vi "Troubleshoot 1.vi"(8 "error in (no error)":errorcluster, 9 "Network Settings in":T6, 10 "Targets in":T1 {"Filtered Targets"."IP Mode" items=["Static"=1, "DHCP/Link-Local"=2, "Link-Local Only"=4, "DHCP Only"=8]}, 11 "Ctl Refs in":T7) -> (0 "error out":errorcluster, 1 "Network Settings out":T6, 2 "Targets out":T1 {"Filtered Targets"."IP Mode" items=["Static"=1, "DHCP/Link-Local"=2, "Link-Local Only"=4, "DHCP Only"=8]}, 3 "Ctl Refs out":T7, 4 "Buttons out":T5, 5 "Execution State":T4, 7 "Deploy out":enum16{"Deploy", "Troubleshoot"}(ring))   [LabVIEW 2013]
uses:
  Controls/Refs.ctl
  Controls/Button Refs.ctl
  Controls/Tab Ctl Refs.ctl
  types/TabStateType.ctl
  Controls/Indicator Refs.ctl
  Controls/Slider Refs.ctl
  Controls/Control Refs.ctl
  Controls/Targets.ctl
  Controls/Detected.ctl
  types/MAX Sys Cfg Target Information.ctl
  Controls/Network Settings.ctl
  types/ButtonStateType.ctl
  types/ExecutionStateType.ctl
panel:
  in  "stop_loop":bool
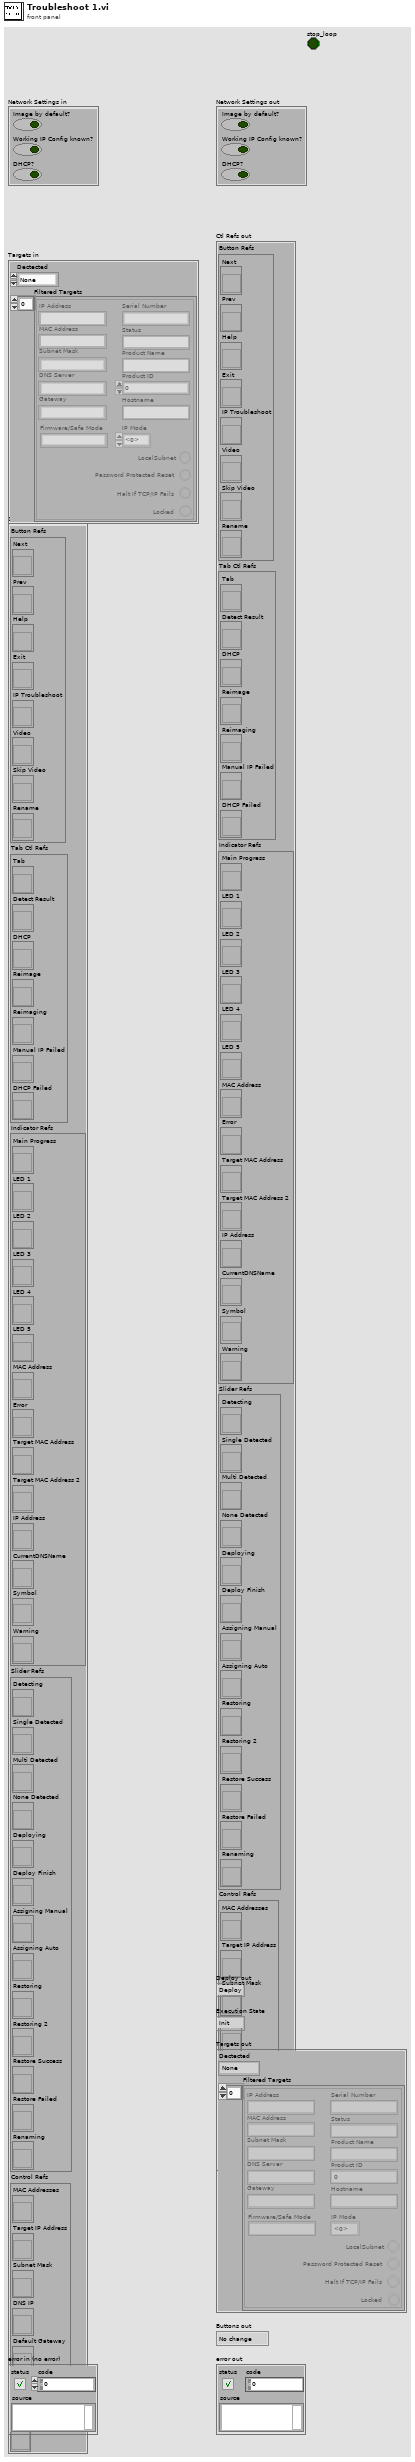
[diagram p1: front panel]
types:
  T1 = typedef "Targets.ctl" = cluster{"Dectected":T2, "Filtered Targets":T3[]}
  T2 = typedef "Detected.ctl" = enum16{"None", "Failed", "Single", "Multi"}
  T3 = typedef "MAX Sys Cfg Target Information.ctl" = cluster{"MAC Address":string, "IP Address":string, "Status":string, "Product Name":string, "Hostname":string, "Firmware/Safe Mode":string, "Subnet Mask":string, "Gateway":string, "DNS Server":string, "Serial Number":string, "Product ID":u32, "Locked ":bool, "LocalSubnet":bool, "Halt If TCP/IP Fails":bool, "Password Protected Reset":bool, "IP Mode":i32}
  T4 = typedef "ExecutionStateType.ctl" = enum16{"Init", "Welcome", "Idle", "Detect", "Run Detection", "Detect Fail", "Detect One", "Detect Mult", "Deploy", "DHCP", "Static IP", "Run Deployment", "Connect Verify", "Exit", "Video Wait", "Success", "Troubleshoot", "Troubleshoot 2", "RenameDNS"}
  T5 = typedef "ButtonStateType.ctl" = enum16{"No change", "No Next", "No Prev", "All Disabled", "All Enabled", "Exit Only"}
  T6 = typedef "Network Settings.ctl" = cluster{"Image by default?":bool, "Working IP Config known?":bool, "DHCP?":bool}
  T7 = typedef "Refs.ctl" = cluster{"Button Refs":T8, "Tab Ctl Refs":T9, "Indicator Refs":T10, "Slider Refs":T11, "Control Refs":T12, "Deploy Message":refnum<vi>}
  T8 = typedef "Button Refs.ctl" = cluster{"Next":refnum<vi>, "Prev":refnum<vi>, "Help":refnum<vi>, "Exit":refnum<vi>, "IP Troubleshoot":refnum<vi>, "Video":refnum<vi>, "Skip Video":refnum<vi>, "Rename":refnum<vi>}
  T9 = typedef "Tab Ctl Refs.ctl" = cluster{"Tab":refnum<vi>, "Detect Result":refnum<vi>, "DHCP":refnum<vi>, "Reimage":refnum<vi>, "Reimaging":refnum<vi>, "Manual IP Failed":refnum<vi>, "DHCP Failed":refnum<vi>}
  T10 = typedef "Indicator Refs.ctl" = cluster{"Main Progress":refnum<vi>, "LED 1":refnum<vi>, "LED 2":refnum<vi>, "LED 3":refnum<vi>, "LED 4":refnum<vi>, "LED 5":refnum<vi>, "MAC Address":refnum<vi>, "Error":refnum<vi>, "Target MAC Address":refnum<vi>, "Target MAC Address 2":refnum<vi>, "IP Address":refnum<vi>, "CurrentDNSName":refnum<vi>, "Symbol":refnum<vi>, "Warning":refnum<vi>}
  T11 = typedef "Slider Refs.ctl" = cluster{"Detecting":refnum<vi>, "Single Detected":refnum<vi>, "Multi Detected":refnum<vi>, "None Detected":refnum<vi>, "Deploying":refnum<vi>, "Deploy Finish":refnum<vi>, "Assigning Manual":refnum<vi>, "Assigning Auto":refnum<vi>, "Restoring":refnum<vi>, "Restoring 2":refnum<vi>, "Restore Success":refnum<vi>, "Restore Failed":refnum<vi>, "Renaming":refnum<vi>}
  T12 = typedef "Control Refs.ctl" = cluster{"MAC Addresses":refnum<vi>, "Target IP Address":refnum<vi>, "Subnet Mask":refnum<vi>, "DNS IP":refnum<vi>, "Default Gateway":refnum<vi>, "DNSName":refnum<vi>}
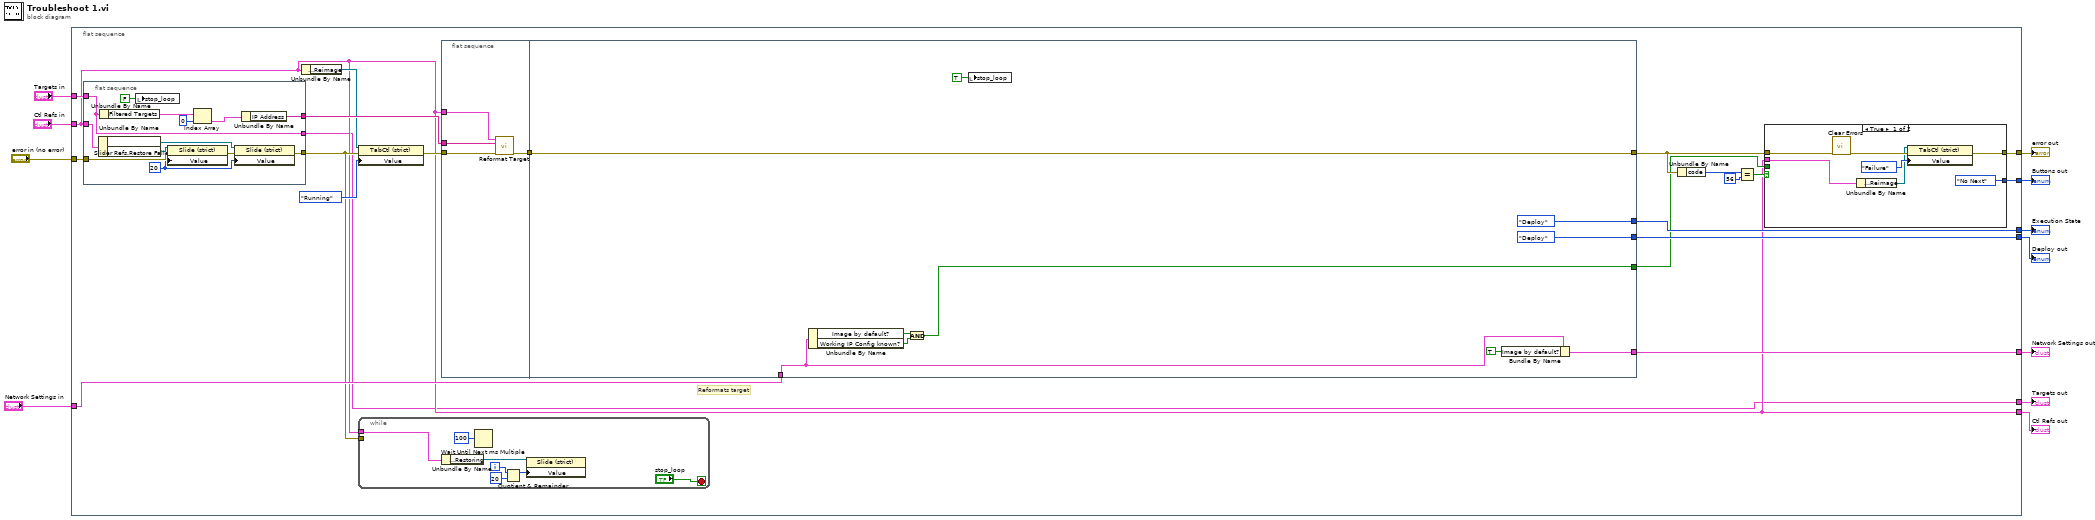
[diagram p0: block diagram]
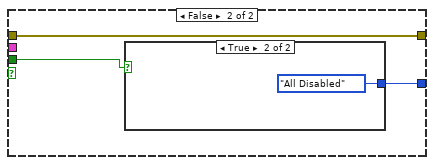
[diagram p2: hidden frame]
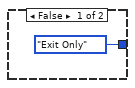
[diagram p3: hidden frame]
diagram:
  n1 = flat-sequence {
    tunnel: "Targets in" -> [w31]
    tunnel: "error in (no error)" -> [w30]
    tunnel: [w26] -> w3
    tunnel: [w25] -> w4
    tunnel: [w20] -> w5
    tunnel: [w19] -> w6
    tunnel: "Network Settings in" -> [w18]
    tunnel: [w15] -> w8
    tunnel: [w12] -> w9
    tunnel: "Ctl Refs in" -> [w13]
    tunnel: [w13] -> w11
    frame #0 {
      # "Reformats target"
      n2 = flat-sequence {
        tunnel: w31 -> [w75]
        tunnel: [w75] -> w12
        tunnel: [w67] -> w16
        tunnel: w30 -> [w73]
        tunnel: [w76] -> w27
        tunnel: w13 -> [w70]
        frame #0 {
          w71 = i8 20 ("Slide 9")
          n3 = Unbundle By Name(w70) -> ("Slider Refs.Restore Success"=w68:refnum<vi>, "Slider Refs.Restore Failed"=w69:refnum<vi>)
          n4 = Unbundle By Name(w75) -> ("Filtered Targets"=w74:T3[])
          n5 = local write "stop_loop"(FALSE ("stop_loop")) -> ()
          n6 = property on="Property Node" class="Slide (strict)"(reference=w69, error in=w73, "Value"=w71) -> (error out=w72:errorcluster)  [unwired: 1 out]
          n7 = Index Array(array=w74, index=0) -> (element=w77:T3)
          n8 = property on="Property Node" class="Slide (strict)"(reference=w68, error in=w72, "Value"=w71) -> (error out=w67:errorcluster)  [unwired: 1 out]
          n9 = Unbundle By Name(w77) -> ("IP Address"=w76:string)
        }
      }
      n10 = Unbundle By Name(w13) -> ("Tab Ctl Refs.Reimage"=w14:refnum<vi>)
      n11 = property on="Property Node" class="TabCtl (strict)"(reference=w14, error in=w16, "Value"=enum32{"Running", "Success", "Failure"}."Running" ("Reimage Tabs")) -> (error out=w28:errorcluster)  [unwired: 1 out]
      n12 = while {
        tunnel: w16 -> [_]
        tunnel: w13 -> [w36]
        i -> [w37]
        stop <- "stop_loop" stop-if-true
        n13 = Unbundle By Name(w36) -> ("Slider Refs.Restoring"=w35:refnum<vi>)
        n14 = Wait Until Next ms Multiple(millisecond multiple=u32 100 ("milliseconds to wait")) -> ()  [unwired: 1 out]
        n15 = Quotient & Remainder(x=w37, y=20) -> (x-y*floor(x/y)=w34:i32)  [unwired: 1 out]
        n16 = property on="Property Node" class="Slide (strict)"(reference=w35, "Value"=w34) -> ()  [unwired: 1 in, 2 out]
      }
      n17 = flat-sequence {
        tunnel: w28 -> [w55]
        tunnel: w27 -> [w53]
        tunnel: [w54] -> w32
        tunnel: w13 -> [w52]
        tunnel: w32 -> [w63]
        tunnel: [ExecutionStateType."Deploy" ("Enum")] -> w26
        tunnel: [w63] -> w21
        tunnel: [enum16{"Deploy", "Troubleshoot"}."Deploy"] -> w25
        tunnel: w18 -> [w60]
        tunnel: [w57] -> w17
        tunnel: [w58] -> w15
        frame #0 {
          n18 = call "Reformat Target.vi"("error in (no error)"=w55, "IP Address"=w53, "Ctl Refs in"=w52) -> ("error out"=w54:errorcluster)  [unwired: 7 in, 1 out]
        }
        frame #1 {
          n19 = Unbundle By Name(w60) -> ("Image by default?"=w61:bool, "Working IP Config known?"=w62:bool)
          n20 = And(x=w61, y=w62) -> (x .and. y?=w57:bool)
          n21 = local write "stop_loop"(TRUE ("stop_loop")) -> ()
          n22 = Bundle By Name(cluster=w60, "Image by default?"=TRUE) -> (w58:T6)
        }
      }
      n23 = Unbundle By Name(w21) -> ("code"=w24:i32)
      n24 = Equal?(x=w24, y=56) -> (x = y?=w22:bool)
      n25 = case shown="True" w22 {
        tunnel: w21 -> [w44 w49]
        tunnel: [w45 w49] -> w20
        tunnel: [ButtonStateType."No Next" ("Enum") w48] -> w19
        tunnel: w17 -> [_ w47]
        tunnel: w13 -> [w40 _]
        frame True {
          n26 = call <vilib>:"Clear Errors.vi"("error in (no error)"=w44) -> ("error out"=w43:errorcluster)  [unwired: 6 out]
          n27 = Unbundle By Name(w40) -> ("Tab Ctl Refs.Reimage"=w41:refnum<vi>)
          n28 = property on="Property Node" class="TabCtl (strict)"(reference=w41, error in=w43, "Value"=enum32{"Running", "Success", "Failure"}."Failure" ("Reimage Tabs")) -> (error out=w45:errorcluster)  [unwired: 1 out]
        }
        frame False {
          n29 = case shown="True" w47 {
            tunnel: [ButtonStateType."Exit Only" ("Enum") ButtonStateType."All Disabled" ("Enum")] -> w48
            frame False {
            }
            frame True {
            }
          }
        }
      }
    }
  }
  "Ctl Refs out" <- w11
  "Targets out" <- w9
  "Network Settings out" <- w8
  "Buttons out" <- w6
  "error out" <- w5
  "Deploy out" <- w4
  "Execution State" <- w3
